vi "Write model_name.vi"(8 "error in (no error)":errorcluster, 10 "model_name":string(combo)="claude-3-5-sonnet-20240620", 11 "llm_anthropic_chatmodels in":refnum<class "llm_anthropic_chatmodels.lvclass">) -> (0 "error out":errorcluster, 3 "llm_anthropic_chatmodels out":refnum<class "llm_anthropic_chatmodels.lvclass">)   [LabVIEW 2020, in "llm_anthropic_chatmodels.lvclass"]
uses:
  llm_anthropic_chatmodels.lvclass
  llm_anthropic_chatmodels.lvclass/llm_anthropic_chatmodels.ctl
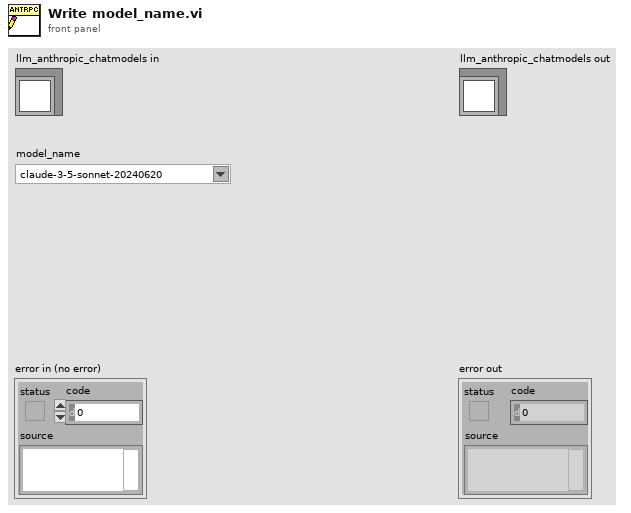
[diagram p1: front panel]
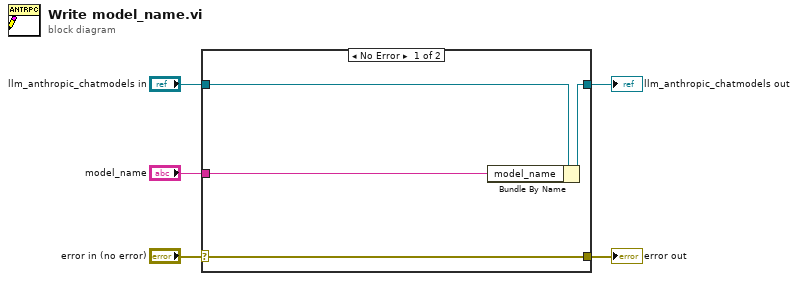
[diagram p0: block diagram]
diagram:
  n1 = case shown="No Error" "error in (no error)" {
    selector: "error in (no error)" -> [w9 w10]
    tunnel: [w9 w10] -> w4
    tunnel: [w7 w11] -> w2
    tunnel: "llm_anthropic_chatmodels in" -> [w8 w11]
    tunnel: "model_name" -> [w6 _]
    frame No Error {
      n2 = Bundle By Name(cluster=w8, "model_name"=w6) -> (w7:refnum<class "llm_anthropic_chatmodels.lvclass">)
    }
    frame Error {
    }
  }
  "error out" <- w4
  "llm_anthropic_chatmodels out" <- w2
